vi "PXI-2514 Channel Page.vi"(8 "error in (no error)":errorcluster, 11 "Node Ptr":T2 format="%.0x") -> (0 "error out":errorcluster)   [LabVIEW 2020, in "PXI-2514 System Explorer.lvlib"]
uses:
  PXI-2514 System Explorer.lvlib
  <vilib>/NI VeriStand/Custom Device API/Custom Device Item Ref.ctl
  Types/Channel Fault Selector.ctl
  Shared/Constants.vi
  <vilib>/NI VeriStand/Custom Device API/Get Item Property (U16).vi
  <vilib>/NI VeriStand/Custom Device API/Custom Device API.lvlib
  Shared/PXI-2514 Shared.lvlib
panel:
  out "Hardware Channel #":u16
  in  "Channel Fault Selector Default Value":T1
  in  "Header":cluster{"Section Name":string}={"Section Name"="Custom Device Item Settings"}
  in  "Description":string
  in  "Name (Alias)":string
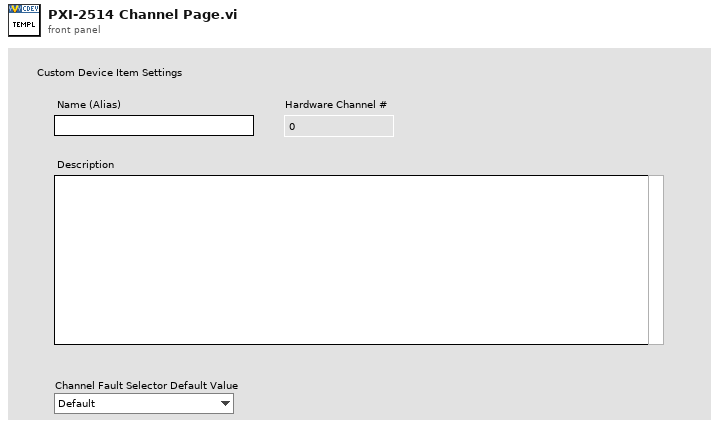
[diagram p1: front panel]
types:
  T1 = typedef "PXI-2514 System Explorer.lvlib/Channel Fault Selector.ctl" = enum16{"Default", "DUT Pass Through", "DUT Open", "DUT Pass Through and FB A", "DUT Pass Through and FB B", "DUT FB A", "DUT FB B"}
  T2 = typedef "Custom Device API.lvlib/Custom Device Item Ref.ctl" = u64
  T3 = typedef "Custom Device API.lvlib/Custom Device Item Info.ctl" = cluster{"Name":string, "Is Channel":bool, "GUID":string, "Is Waveform":bool}
  T4 = typedef "Custom Device API.lvlib/Custom Device Channel.ctl" = cluster{"Type":T5, "Units":string, "Default Value":dbl, "Faultable":bool, "Scalable":bool}
  T5 = typedef "Custom Device API.lvlib/Custom Device Channel Type.ctl" = enum16{"Input", "Output"}
  T6 = typedef "Custom Device API.lvlib/Custom Device Commands.ctl" = enum16{"Default", "Item renamed", "Shutdown", "Dynamic button pressed"}
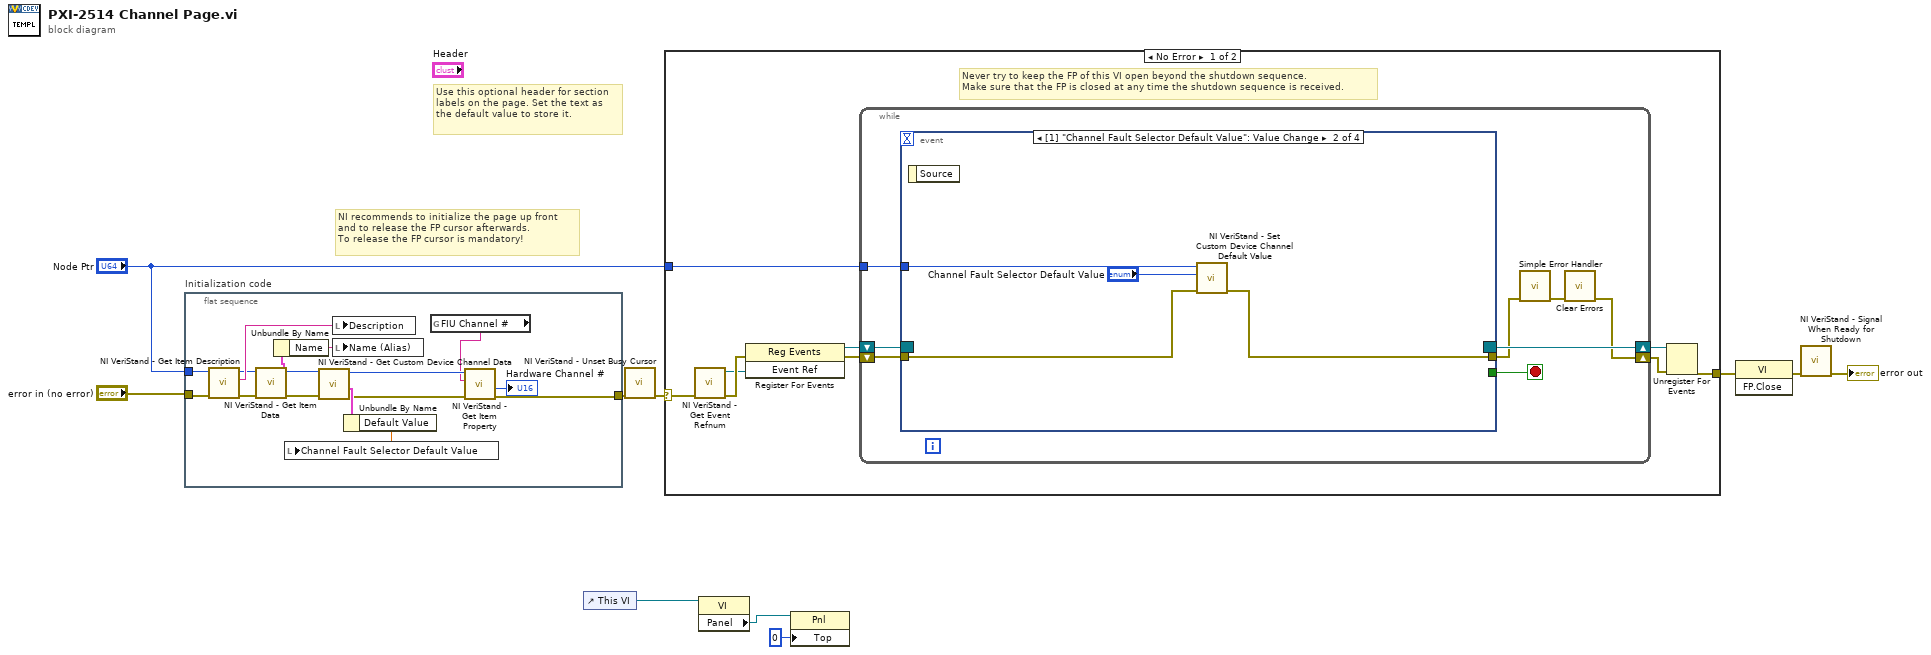
[diagram p0: block diagram]
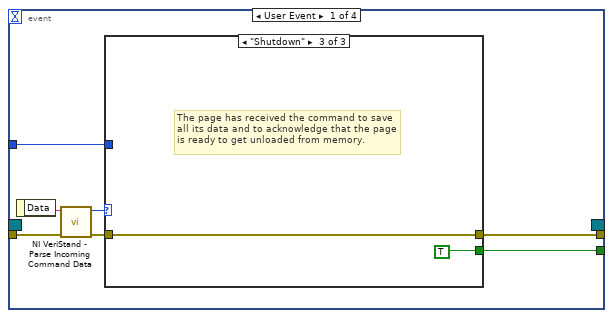
[diagram p2: hidden frame]
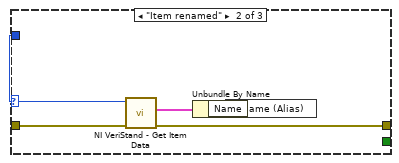
[diagram p4: hidden frame]
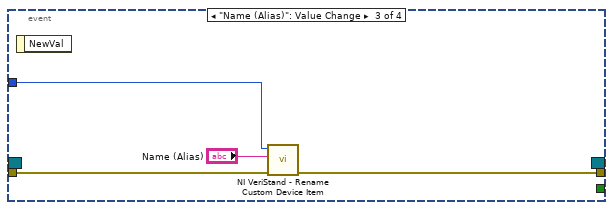
[diagram p5: hidden frame]
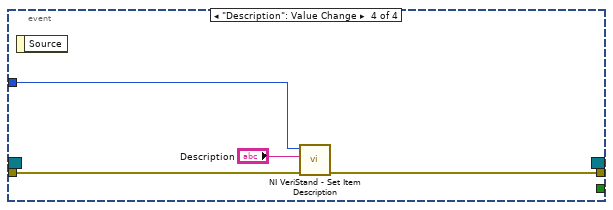
[diagram p6: hidden frame]
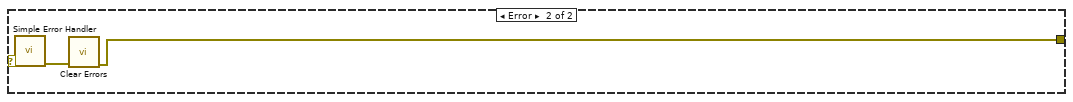
[diagram p7: hidden frame]
diagram:
  # "Use this optional header for section labels on the page. Set the text as the default value to store it."
  # "NI recommends to initialize the page up front\nand to release the FP cursor afterwards.\nTo release the FP cursor is mandatory!"
  n1 = flat-sequence "Initialization code" {
    tunnel: "error in (no error)" -> [w26]
    tunnel: "Node Ptr" -> [w25]
    tunnel: [w12] -> w6
    frame #0 {
      n2 = call <vilib>:"NI VeriStand - Get Item Description.vi"("error in (no error)"=w26, "Item Ref in"=w25) -> ("error out"=w23:errorcluster, "Description"=w24:string, "Item Ref out"=w22:T2)  [unwired: 7 out]
      n3 = call <vilib>:"NI VeriStand - Get Item Data.vi"("error in (no error)"=w23, "Item Ref in"=w22) -> ("error out"=w18:errorcluster, "Item Info"=w21:T3, "Item Ref out"=w19:T2)  [unwired: 7 out]
      n4 = Unbundle By Name(w21) -> ("Name"=w20:string)
      n5 = call <vilib>:"NI VeriStand - Get Custom Device Channel Data.vi"("error in (no error)"=w18, "Channel Ref in"=w19) -> ("error out"=w14:errorcluster, "Channel"=w17:T4, "Channel Ref out"=w15:T2)  [unwired: 4 in, 3 out]
      n6 = local write "Description"(w24) -> ()
      n7 = local write "Name (Alias)"(w20) -> ()
      n8 = Unbundle By Name(w17) -> ("Default Value"=w16:dbl)
      n9 = local write "Channel Fault Selector Default Value"(w16) -> ()
      n10 = global read "Constants.vi" "FIU Channel #"() -> (w11:string)
      n11 = call-poly <vilib>:"NI VeriStand - Get Item Property.vi"("error in (no error)"=w14, "Property Name"=w11, "Item Ref in"=w15) -> ("error out"=w12:errorcluster, "Value"=→"Hardware Channel #":u16)  [unwired: 5 in, 2 out]
    }
  }
  n12 = control-ref of="This VI"() -> (w3:refnum<vi>)
  n13 = call <vilib>:"NI VeriStand - Unset Busy Cursor.vi"("error in (no error)"=w6) -> ("error out"=w5:errorcluster)  [unwired: 10 out]
  n14 = case shown="No Error" w5 {
    selector: w5 -> [w27 w73]
    tunnel: [w32 w71] -> w10
    tunnel: "Node Ptr" -> [w28 _]
    frame No Error {
      # "Never try to keep the FP of this VI open beyond the shutdown sequence.\nMake sure that the FP is closed at any time the shutdown sequence is received."
      n15 = call <vilib>:"NI VeriStand - Get Event Refnum.vi"("error in (no error)"=w27) -> ("error out"=w35:errorcluster, "Event Ref"=w31:refnum<user-event>)  [unwired: 9 out]
      n16 = register-events(error in=w35, w31) -> (reference out=w29:refnum<event-registration>, error out=w30:errorcluster)  [unwired: 1 in]
      n17 = while {
        tunnel: w28 -> [w39]
        shift-right: [w36] -> w33
        shift-left: w30 -> [w42]
        shift-right: [w43] -> w34
        shift-left: w29 -> [w41]
        stop <- w40 stop-if-true
        n18 = event shown="[1] \"Channel Fault Selector Default Value\": Value Change" {
          selector: w41 -> [_ _ _ _]
          dyn-events: [_ _ _ _] -> w43
          timeout: _ -> [_ _ _ _]
          tunnel: w42 -> [w50 w60 w66 w69]
          tunnel: [w46 _ _ _] -> w40
          tunnel: [w45 w59 w65 w68] -> w38
          tunnel: w39 -> [w44 w62 w64 w70]
          event User Event {
            n19 = event-data() -> ("Data"=w49:string)  [unwired: 1 out]
            n20 = call <vilib>:"NI VeriStand - Parse Incoming Command Data.vi"("error in (no error)"=w50, "Incoming data"=w49) -> ("error out"=w48:errorcluster, "Action"=w47:T6)  [unwired: 8 out]
            n21 = case shown="\"Shutdown\"" w47 {
              tunnel: w48 -> [w51 w56 w57]
              tunnel: [_ _ TRUE] -> w46
              tunnel: [w51 w53 w57] -> w45
              tunnel: w44 -> [_ w55 _]
              frame "Default", Default {
              }
              frame "Item renamed" {
                n22 = call <vilib>:"NI VeriStand - Get Item Data.vi"("error in (no error)"=w56, "Item Ref in"=w55) -> ("error out"=w53:errorcluster, "Item Info"=w54:T3)  [unwired: 8 out]
                n23 = Unbundle By Name(w54) -> ("Name"=w52:string)
                n24 = local write "Name (Alias)"(w52) -> ()
              }
              frame "Shutdown" {
                # "The page has received the command to save all its data and to acknowledge that the page is ready to get unloaded from memory."
              }
            }
          }
          event Value Change {
            n25 = event-data() -> ()  [unwired: 2 out]
            n26 = call <vilib>:"NI VeriStand - Set Custom Device Channel Default Value.vi"("error in (no error)"=w60, "Default Value"="Channel Fault Selector Default Value", "Channel Ref in"=w62) -> ("error out"=w59:errorcluster)  [unwired: 7 in, 1 out]
          }
          event "Name (Alias)": Value Change {
            n27 = event-data() -> ()  [unwired: 2 out]
            n28 = call <vilib>:"NI VeriStand - Rename Custom Device Item.vi"("error in (no error)"=w66, "New Name"="Name (Alias)", "Item Ref in"=w64) -> ("error out"=w65:errorcluster)  [unwired: 1 in, 7 out]
          }
          event "Description": Value Change {
            n29 = event-data() -> ()  [unwired: 2 out]
            n30 = call <vilib>:"NI VeriStand - Set Item Description.vi"("error in (no error)"=w69, "Description"="Description", "Item Ref in"=w70) -> ("error out"=w68:errorcluster)  [unwired: 8 out]
          }
        }
        n31 = call <vilib>:"Simple Error Handler.vi"("error in (no error)"=w38) -> ("error out"=w37:errorcluster)  [unwired: 1 in, 7 out]
        n32 = call <vilib>:"Clear Errors.vi"("error in (no error)"=w37) -> ("error out"=w36:errorcluster)  [unwired: 1 in, 5 out]
      }
      n33 = Unregister For Events(event registration refnum=w34, error in=w33) -> (error out=w32:errorcluster)
    }
    frame Error {
      n34 = call <vilib>:"Simple Error Handler.vi"("error in (no error)"=w73) -> ("error out"=w72:errorcluster)  [unwired: 1 in, 7 out]
      n35 = call <vilib>:"Clear Errors.vi"("error in (no error)"=w72) -> ("error out"=w71:errorcluster)  [unwired: 1 in, 5 out]
    }
  }
  n36 = property class="VI"(reference=w3) -> ("Panel"=w2:refnum<vi>)  [unwired: 1 in, 2 out]
  n37 = property class="Pnl"(reference=w2, "Top"=0 ("Position:Top")) -> ()  [unwired: 1 in, 2 out]
  n38 = invoke class="VI" method="FP.Close"(error in=w10) -> (error out=w9:errorcluster)  [unwired: 2 in, 2 out]
  n39 = call <vilib>:"NI VeriStand - Signal When Ready for Shutdown.vi"("error in (no error)"=w9) -> ("error out"=→"error out":errorcluster)  [unwired: 10 out]
